vi "RSZVB Load Port Pair Circuit Model Data.vi"(4 "Interchange Port Numbers (Off)":bool, 5 "Parameter (Port 1)":i32(ring) items=["Port 1", "Port 2"], 6 "File Name (\"\")":string, 7 "Port Pair (1)":i32=1, 8 "error in (no error)":errorcluster {"code" format="%.0x"}, 9 "Function Type (Deembedding)":i32(ring) items=["Deembedding", "Embedding"], 10 "Channel (1)":i32=1, 11 "VISA session":refnum<visa-resource-name>) -> (0 "error out":errorcluster {"code" format="%.0x"}, 3 "dup VISA session":refnum<visa-resource-name>)   [LabVIEW 2011]
doc: "This VI loads data from a specified Touchstone file defining the characteristics of the current embedded/deembedded port pair circuit model. A balanced port circuit model involving file import must be selected before using this VI. \n\nRemote-control command(s):\nMMEMory:LOAD:VNETworks<Ch>:PPAir:EMBedding<List_idx> '<file_name>', PMAin | PSECondary \nMMEMory:LOAD:VNETworks<Ch>:PPAir:DEEMbedding<List_idx> '<file_name>', PMAin | PSECondary"
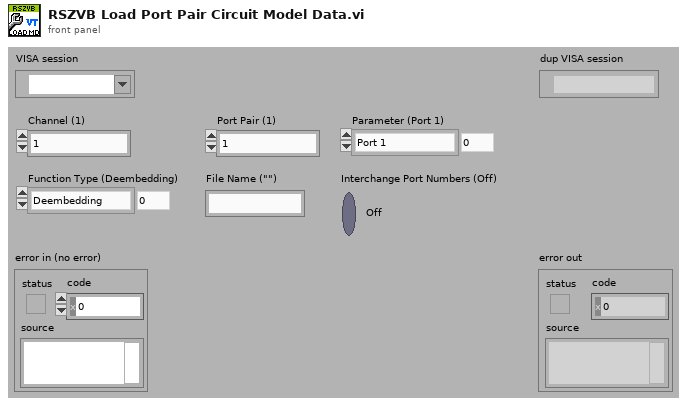
[diagram p1: front panel]
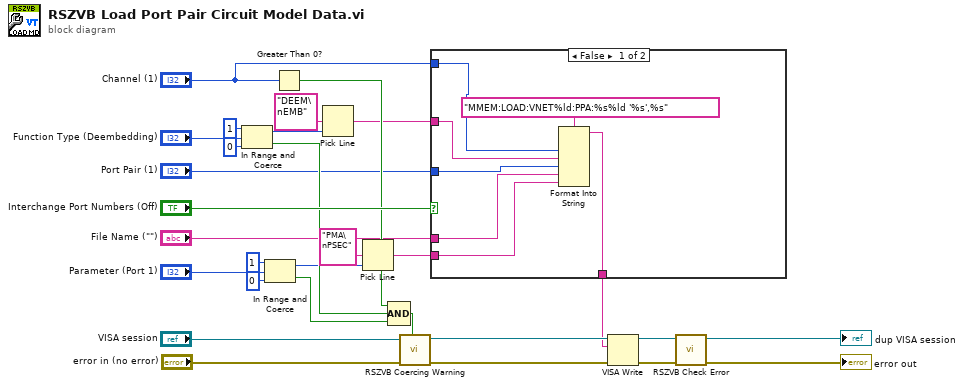
[diagram p0: block diagram]
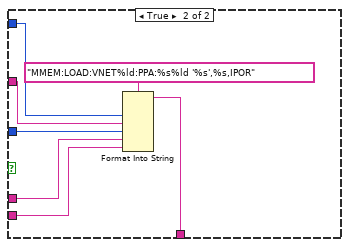
[diagram p2: hidden frame]
diagram:
  n1 = In Range and Coerce(upper limit=1, x="Function Type (Deembedding)", lower limit=0) -> (coerced(x)=w26:i32, In Range?=w19:bool)
  n2 = In Range and Coerce(upper limit=1, x="Parameter (Port 1)", lower limit=0) -> (coerced(x)=w2:i32, In Range?=w10:bool)
  n3 = Greater Than 0?(x="Channel (1)") -> (x > 0?=w18:bool)
  n4 = Pick Line(multi-line string="DEEM\nEMB", line index=w26) -> (output string=w16:string)  [unwired: 1 in]
  n5 = Pick Line(multi-line string="PMA\nPSEC", line index=w2) -> (output string=w1:string)  [unwired: 1 in]
  n6 = Compound Arithmetic op=AND(w18, w19, w10) -> (w22:bool)
  n7 = call "RSZVB Coercing Warning.vi"("In Range?"=w22, "error in (no error)"="error in (no error)", "VISA session"="VISA session") -> ("error out"=w23:errorcluster, "dup VISA session"=w24:refnum<visa-resource-name>)  [unwired: 7 in]
  n8 = case shown="False" "Interchange Port Numbers (Off)" {
    tunnel: [w30 w42] -> w21
    tunnel: "Channel (1)" -> [w35 w41]
    tunnel: w16 -> [w34 w40]
    tunnel: "Port Pair (1)" -> [w33 w39]
    tunnel: "File Name (\"\")" -> [w32 w38]
    tunnel: w1 -> [w31 w37]
    frame False {
      n9 = Format Into String(format string="MMEM:LOAD:VNET%ld:PPA:%s%ld '%s',%s", w35, w34, w33, w32, w31) -> (resulting string=w30:string)  [unwired: 2 in, 1 out]
    }
    frame True {
      n10 = Format Into String(format string="MMEM:LOAD:VNET%ld:PPA:%s%ld '%s',%s,IPOR", w41, w40, w39, w38, w37) -> (resulting string=w42:string)  [unwired: 2 in, 1 out]
    }
  }
  n11 = VISA Write(VISA resource name=w24, write buffer=w21, error in (no error)=w23) -> (VISA resource name out=w7:refnum<visa-resource-name>, error out=w6:errorcluster)  [unwired: 1 out]
  n12 = call "RSZVB Check Error.vi"("error in (no error)"=w6, "VISA session"=w7) -> ("error out"=→"error out":errorcluster, "dup VISA session"=→"dup VISA session":refnum<visa-resource-name>)  [unwired: 8 in]
